vi "multi_data_output.vi"() -> ()   [LabVIEW 2017]
panel:
  out "Running":bool
  in  "stop (F)":bool
  in  "Waveform Path":path
  # "This vi takes a .csv file as input and uses the 8 channels to output via analog output"
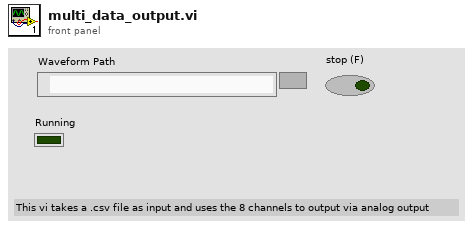
[diagram p1: front panel]
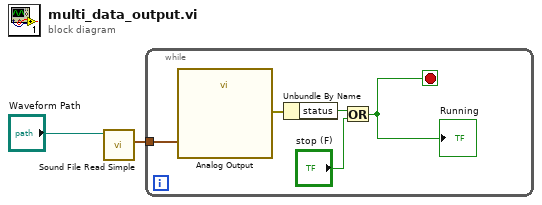
[diagram p0: block diagram]
diagram:
  n1 = call <vilib>:"Sound File Read Simple.vi"("path"="Waveform Path") -> ("data"=w2:waveform(dbl)[])  [unwired: 7 in, 3 out]
  n2 = while {
    tunnel: w2 -> [w7]
    stop <- w3 stop-if-true
    n3 = call "Analog Output"("data"=w7) -> ("error out"=w6:errorcluster)  [unwired: 16 in, 2 out]
    n4 = Unbundle By Name(w6) -> ("status"=w4:bool)
    n5 = Or(x=w4, y="stop (F)") -> (x .or. y?=w3:bool)
    "Running" <- w3
  }
